vi "Cmd_U32U32U32U32.vi"(4 "Arg3":u32, 5 "Arg2":u32 max=127 step=1, 6 "Arg4":u32, 7 "Arg1":u32 max=127 step=1, 8 "error in (no error)":errorcluster, 9 "Cmd":u8, 10 "Address":u8, 11 "VISA Refnum in":refnum<visa-resource-name>) -> (0 "error out":errorcluster, 2 "Valid":bool, 3 "VISA Refnum out":refnum<visa-resource-name>)   [LabVIEW 2015, in "Ion Motion Roboclaw.lvlib"]
uses:
  <instrlib>/Ion Motion Roboclaw/Ion Motion Roboclaw.lvlib
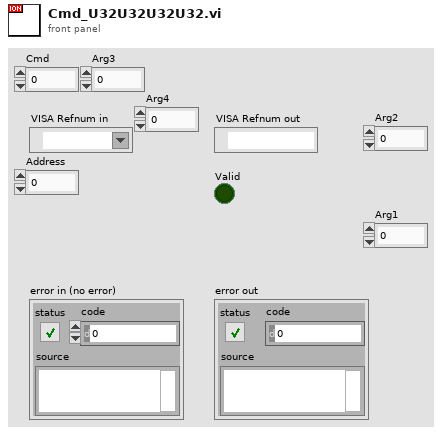
[diagram p1: front panel]
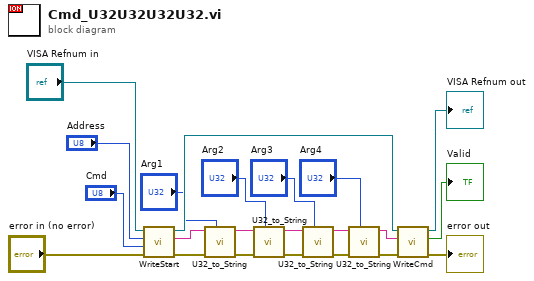
[diagram p0: block diagram]
diagram:
  n1 = call <instrlib>:"WriteStart.vi"("error in (no error)"="error in (no error)", "Cmd"="Cmd", "Address"="Address", "VISA Refnum in"="VISA Refnum in") -> ("error out"=w14:errorcluster, "String Out"=w15:string, "VISA Refnum out"=w17:refnum<visa-resource-name>)  [unwired: 5 in]
  n2 = call <instrlib>:"U32_to_String.vi"("number"="Arg1", "error in (no error)"=w14, "String In"=w15) -> ("error out"=w13:errorcluster, "String Out"=w12:string)  [unwired: 5 in]
  n3 = call <instrlib>:"U32_to_String.vi"("number"="Arg2", "error in (no error)"=w13, "String In"=w12) -> ("error out"=w7:errorcluster, "String Out"=w8:string)  [unwired: 5 in]
  n4 = call <instrlib>:"U32_to_String.vi"("number"="Arg3", "error in (no error)"=w7, "String In"=w8) -> ("error out"=w5:errorcluster, "String Out"=w3:string)  [unwired: 5 in]
  n5 = call <instrlib>:"U32_to_String.vi"("number"="Arg4", "error in (no error)"=w5, "String In"=w3) -> ("error out"=w4:errorcluster, "String Out"=w2:string)  [unwired: 5 in]
  n6 = call <instrlib>:"WriteCmd.vi"("error in (no error)"=w4, "write buffer"=w2, "VISA Refnum in"=w17) -> ("error out"=→"error out":errorcluster, "Valid"=→"Valid":bool, "VISA Refnum out"=→"VISA Refnum out":refnum<visa-resource-name>)  [unwired: 2 in]
